vi "FRIC_navX_Get_YPRHfH.vi"(6 "Zero":bool, 7 "Update":bool) -> (2 "YRPHfH":T1)   [LabVIEW 2015, in "navX AE v1.lvlib"]
doc: "This navX VI returns the Yaw, Roll, Pitch, Heading, Fused Heading of the navX."
uses:
  navX AE v1.lvlib
  navX Library v2/_TypeDefs/Z900_navX_DeviceRegisters.ctl
  navX Library v2/navX Library v2.lvlib
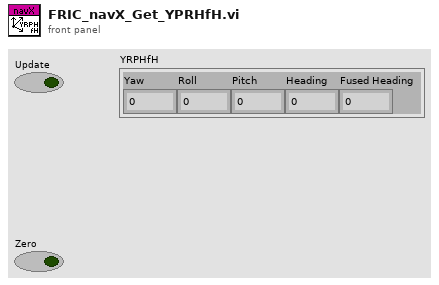
[diagram p1: front panel]
types:
  T1 = cluster{"Yaw":dbl, "Roll":dbl, "Pitch":dbl, "Heading":dbl, "Fused Heading":dbl}
  T2 = typedef "navX Library v2.lvlib/Z900_navX_DeviceRegisters.ctl" = u8
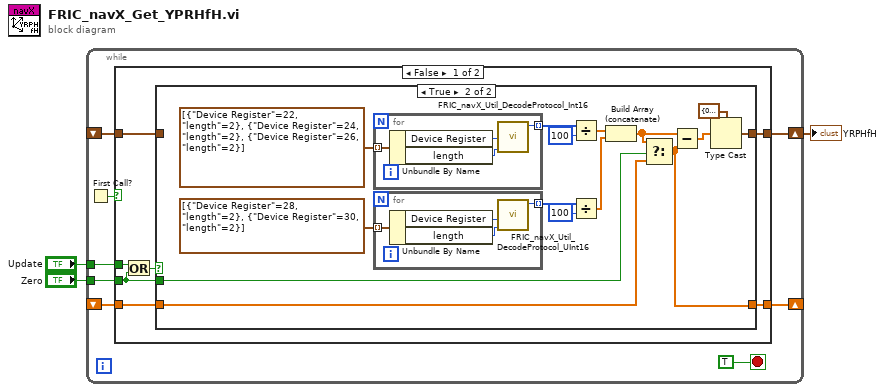
[diagram p0: block diagram]
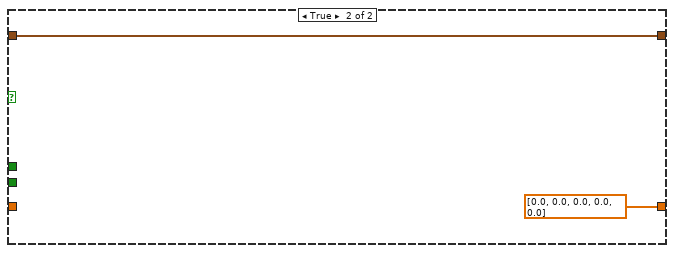
[diagram p3: hidden frame]
diagram:
  n1 = while {
    shift-right: [w9] -> w3
    shift-left: _ -> [w10]
    tunnel: "Update" -> [w8]
    shift-right: [w6] -> _
    shift-left: _ -> [w7]
    tunnel: "Zero" -> [w5]
    stop <- TRUE stop-if-true
    n2 = First Call?() -> (First Call?: T/F=w4:bool)
    n3 = case shown="False" w4 {
      tunnel: w10 -> [w18 w45]
      tunnel: [w17 w45] -> w9
      tunnel: w8 -> [w14 _]
      tunnel: w7 -> [w16 _]
      tunnel: [w15 dbl[] [0.0, 0.0, 0.0, 0.0, 0.0] ("f")] -> w6
      tunnel: w5 -> [w13 _]
      frame False {
        n4 = Or(x=w14, y=w13) -> (x .or. y?=w12:bool)
        n5 = case shown="True" w12 {
          tunnel: [w20 w34] -> w17
          tunnel: w18 -> [w20 _]
          tunnel: w16 -> [w19 w23]
          tunnel: [w19 w22] -> w15
          tunnel: w13 -> [_ w21]
          frame False {
          }
          frame True {
            n6 = for {
              tunnel: cluster{"Device Register":T2, "length":i32}[] [{"Device Register"=22, "length"=2}, {"Device Register"=24, "length"=2}, {"Device Register"=26, "length"=2}] ("Array") -> [w41] mode=indexing
              tunnel: [w40] -> w29 mode=indexing
              n7 = Unbundle By Name(w41) -> ("Device Register"=w43:T2, "length"=w42:i32)
              n8 = call "FRIC_navX_Util_DecodeProtocol_Int16.vi"("length"=w42, "Device Register"=w43) -> ("Value"=w40:i16)  [unwired: 9 in]
            }
            n9 = for {
              tunnel: cluster{"Device Register":T2, "length":i32}[] [{"Device Register"=28, "length"=2}, {"Device Register"=30, "length"=2}] ("Array") -> [w39] mode=indexing
              tunnel: [w36] -> w27 mode=indexing
              n10 = Unbundle By Name(w39) -> ("Device Register"=w38:T2, "length"=w37:i32)
              n11 = call "FRIC_navX_Util_DecodeProtocol_UInt16.vi"("length"=w37, "Device Register"=w38) -> ("Value"=w36:u16)  [unwired: 9 in]
            }
            n12 = Divide(x=w29, y=100) -> (x/y=w26:dbl[])
            n13 = Divide(x=w27, y=100) -> (x/y=w31:dbl[])
            n14 = Build Array (concatenate)(w26, w31) -> (w24:dbl[])
            n15 = Select(t=w24, s=w21, f=w23) -> (s? t:f=w22:dbl[])
            n16 = Subtract(x=w24, y=w22) -> (x-y=w25:dbl[])
            n17 = Type Cast(type=T1 {"Yaw"=0.0, "Roll"=0.0, "Pitch"=0.0, "Heading"=0.0, "Fused Heading"=0.0}, x=w25) -> (*(type *) &x=w34:T1)
          }
        }
      }
      frame True {
      }
    }
  }
  "YRPHfH" <- w3
